vi "poly_is_either_run_state.vi"(4 "execution state":T1(ring)) -> (1 "is running?":bool)   [LabVIEW 2015]
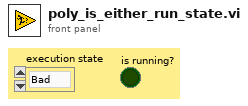
[diagram p1: front panel]
types:
  T1 = enum32{"Bad", "Idle", "Run top level", "Running"}
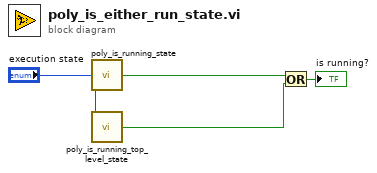
[diagram p0: block diagram]
diagram:
  n1 = call "poly_is_running_state.vi"("execution state"="execution state") -> ("state = 'Running'?"=w3:bool)  [unwired: 4 in]
  n2 = call "poly_is_running_top_level_state.vi"("execution state"="execution state") -> ("state = 'Run top level'?"=w2:bool)  [unwired: 4 in]
  n3 = Or(x=w3, y=w2) -> (x .or. y?=→"is running?":bool)
